vi "HFRR ADV v07 new software.vi"() -> ()   [LabVIEW 2025] (continued)
                        n2281 = local write "EVENT LOG"(w3339) -> ()
                      }
                      frame #26 {
                        n2282 = Wait (ms)(milliseconds to wait=u32 50) -> ()  [unwired: 1 out]
                      }
                      frame #27 {
                        n2283 = local read "Set Temp"() -> (w3343:dbl)
                        n2284 = Number To Fractional String(number=w3343, precision (6)=i16 2) -> (F-format string=w3344:string)  [unwired: 2 in]
                        n2285 = Concatenate Strings("Set Temperature [deg C] :" ("Content"), w3344) -> (w3346:string)
                        n2286 = local read "EVENT LOG"() -> (w3348:string)
                        n2287 = call "Event Log.vi"("Content"=w3346, "EVENT LOG"=w3348) -> ("EVENT LOG"=w3347:string)  [unwired: 8 in, 1 out]
                        n2288 = local write "EVENT LOG"(w3347) -> ()
                      }
                      frame #28 {
                        n2289 = Wait (ms)(milliseconds to wait=u32 50) -> ()  [unwired: 1 out]
                      }
                      frame #29 {
                        n2290 = local read "Set Rh"() -> (w3351:dbl)
                        n2291 = Number To Fractional String(number=w3351, precision (6)=i16 2) -> (F-format string=w3352:string)  [unwired: 2 in]
                        n2292 = Concatenate Strings("Set Humidity [%RH] :" ("Content"), w3352) -> (w3354:string)
                        n2293 = local read "EVENT LOG"() -> (w3356:string)
                        n2294 = call "Event Log.vi"("Content"=w3354, "EVENT LOG"=w3356) -> ("EVENT LOG"=w3355:string)  [unwired: 8 in, 1 out]
                        n2295 = local write "EVENT LOG"(w3355) -> ()
                      }
                      frame #30 {
                        n2296 = Wait (ms)(milliseconds to wait=u32 50) -> ()  [unwired: 1 out]
                      }
                      frame #31 {
                        n2297 = local read "test time"() -> (w3359:dbl)
                        n2298 = Number To Fractional String(number=w3359, precision (6)=i16 1) -> (F-format string=w3360:string)  [unwired: 2 in]
                        n2299 = Concatenate Strings("Test Duration [mins] :" ("Content"), w3360) -> (w3362:string)
                        n2300 = local read "EVENT LOG"() -> (w3364:string)
                        n2301 = call "Event Log.vi"("Content"=w3362, "EVENT LOG"=w3364) -> ("EVENT LOG"=w3363:string)  [unwired: 8 in, 1 out]
                        n2302 = local write "EVENT LOG"(w3363) -> ()
                      }
                      frame #32 {
                        w3365 = dbl[] [] ("History Data")
                        w3366 = cluster{"y":dbl, dbl, "y":dbl}[] [] ("History Data")
                        w3367 = FALSE ("Visible")
                        n2303 = property on="Stroke ( mm )" class="WFChart (strict)"("History Data"=w3366) -> ()  [unwired: 2 in, 2 out]
                        n2304 = property on="Humidity ( %RH )" class="WFChart (strict)"("History Data"=w3365) -> ()  [unwired: 2 in, 2 out]
                        n2305 = property on="Temperature ( Deg C )" class="WFChart (strict)"("History Data"=w3365) -> ()  [unwired: 2 in, 2 out]
                        n2306 = property on="Electrical Contact Resistance ( % )" class="WFChart (strict)"("History Data"=w3365) -> ()  [unwired: 2 in, 2 out]
                        n2307 = property on="Coefficient of Friction" class="WFChart (strict)"("History Data"=w3365) -> ()  [unwired: 2 in, 2 out]
                        n2308 = property on="Frictional Force ( N )" class="WFChart (strict)"("History Data"=w3365) -> ()  [unwired: 2 in, 2 out]
                        n2309 = property on="Coefficient of Friction" class="WFChart (strict)"("History Data"=w3365) -> ()  [unwired: 2 in, 2 out]
                        n2310 = property on="Frictional Force ( N )" class="WFChart (strict)"("History Data"=w3365) -> ()  [unwired: 2 in, 2 out]
                        n2311 = property on="Electrical Contact Resistance ( % )" class="WFChart (strict)"("History Data"=w3365) -> ()  [unwired: 2 in, 2 out]
                        n2312 = property on="Humidity ( %RH )" class="WFChart (strict)"("History Data"=w3365) -> ()  [unwired: 2 in, 2 out]
                        n2313 = property on="Stroke ( mm )" class="WFChart (strict)"("History Data"=w3366) -> ()  [unwired: 2 in, 2 out]
                        n2314 = property on="Temperature ( Deg C )" class="WFChart (strict)"("History Data"=w3365) -> ()  [unwired: 2 in, 2 out]
                        n2315 = property on="Service Password Log" class="Str"("Visible"=w3367) -> ()  [unwired: 2 in, 2 out]
                        n2316 = property on="Password 3" class="Clust (strict)"("Visible"=w3367) -> ()  [unwired: 2 in, 2 out]
                      }
                    }
                    "TEST FILE NAM,E SAVED" <- TRUE ("TEST FILE NAM,E SAVED")
                  }
                }
              }
            }
          }
        }
        n2317 = case shown="True" w2671 {
          frame False {
            n2318 = local write "tfalg"(0.0 ("tfalg")) -> ()
          }
          frame True {
            n2319 = local read "tfalg"() -> (w2816:dbl)
            n2320 = Equal?(x=w2816, y=0.0) -> (x = y?=w2817:bool)
            n2321 = case shown="True" w2817 {
              frame False {
              }
              frame True {
                n2322 = local read "Total No. of Tests"() -> (w2820:dbl)
                n2323 = local write "tfalg"(1.0 ("tfalg")) -> ()
                n2324 = local write "acq 2"(FALSE ("acq 2")) -> ()
                n2325 = Wait (ms)(milliseconds to wait=u32 200) -> ()  [unwired: 1 out]
                n2326 = Increment(x=w2820) -> (x+1=w2819:dbl)
                n2327 = local write "Total No. of Tests"(w2819) -> ()
              }
            }
          }
        }
        n2328 = local write "Test \nStatus"(w2677) -> ()
        n2329 = local write "Save"(w2677) -> ()
        n2330 = local read "Main Tab"() -> (w2634:T2)
        n2331 = case shown="True" w2658 {
          tunnel: [FALSE ("RUN") TRUE ("RUN")] -> w2657
          tunnel: [_ 1] -> w2650
          frame False {
          }
          frame True {
          }
        }
        n2332 = In Range and Coerce(upper limit=w2665, x=w2638, lower limit=w2664) -> (In Range?=w2656:bool)  [unwired: 1 out]
        n2333 = In Range and Coerce(upper limit=w2662, x=w2637, lower limit=w2663) -> (In Range?=w2654:bool)  [unwired: 1 out]
        n2334 = case shown="True" w2670 {
          frame False {
            n2335 = local read "Rt 3"() -> (w2798:bool)
            n2336 = case shown="True" w2798 {
              frame False {
              }
              frame True {
                n2337 = local write "Rt 3"(FALSE ("Rt 3")) -> ()
                n2338 = local write "Json End Flg"(TRUE ("Upld AR 2")) -> ()
              }
            }
            "Rt" <- TRUE ("Rt")
            "Rt 2" <- FALSE ("Rt")
          }
          frame True {
            n2339 = local read "Rt"() -> (w2805:bool)
            n2340 = local write "Rt 2"(TRUE ("Rt 2")) -> ()
            n2341 = case shown="True" w2805 {
              frame False {
              }
              frame True {
                w2806 = TRUE ("Upld AR 2")
                n2342 = local write "Rt"(FALSE ("Rt")) -> ()
                n2343 = local write "Upld AR"(w2806) -> ()
                n2344 = local write "Json St Flg"(w2806) -> ()
              }
            }
            "Rt 3" <- TRUE ("Rt 3")
          }
        }
        n2345 = case shown="True" w2656 {
          tunnel: [FALSE ("RUN") TRUE ("RUN")] -> w2655
          tunnel: [_ 2] -> w2649
          frame False {
          }
          frame True {
          }
        }
        n2346 = case shown="True" w2654 {
          tunnel: [FALSE ("RUN") TRUE ("RUN")] -> w2653
          tunnel: [_ 3] -> w2648
          frame False {
          }
          frame True {
          }
        }
        n2347 = case shown="\"Acquire\"" w2634 {
          tunnel: w2636 -> [_ w2867]
          frame Default {
            w2866 = 0.0 ("output")
            n2348 = local write "PID-out"(w2866) -> ()
            n2349 = local write "Frequency ( Hz )"(w2866) -> ()
          }
          frame "Acquire" {
            n2350 = stacked-sequence {
              frame #0 {
                n2351 = local read "Auto Start Test"() -> (w2869:bool)
                n2352 = case shown="True" w2869 {
                  tunnel: "RUN" -> [w2890 w2893]
                  tunnel: [w2890 w2892] -> w2870
                  frame False {
                  }
                  frame True {
                    n2353 = local read "Auto Start Temp"() -> (w2891:bool)
                    n2354 = Or(x=w2893, y=w2891) -> (x .or. y?=w2892:bool)
                  }
                }
                n2355 = local read "clk"() -> (w2889:dbl)
                n2356 = local read "Save"() -> (w2885:bool)
                n2357 = Equal?(x=w2889, y=0.0) -> (x = y?=w2886:bool)
                n2358 = And(x=w2886, y=w2885) -> (x .and. y?=w2887:bool)
                n2359 = Not(x="Engage") -> (.not. x?=w2876:bool)
                n2360 = case shown="False" w2870 {
                  tunnel: [0.0 w2911] -> w2872
                  frame False {
                    (unwired) TRUE ("Visible")
                    n2361 = local read "Auto Start Test"() -> (w2897:bool)
                    n2362 = local write "Start Time"(TRUE ("Start Time")) -> ()
                    n2363 = property on="Stroke 2" class="DigNum (strict)"("Visible"=FALSE) -> ()  [unwired: 2 in, 2 out]
                    n2364 = case shown="False" w2897 {
                      frame False {
                        n2365 = property on="Heater Button" class="Bool (strict)"("DisabledEnum"=T15."Enabled" ("Disabled")) -> ()  [unwired: 2 in, 2 out]
                        n2366 = property on="Humidity" class="Bool (strict)"("DisabledEnum"=T15."Enabled" ("Disabled")) -> ()  [unwired: 2 in, 2 out]
                      }
                      frame True {
                      }
                    }
                    n2367 = case shown="False" "TestCompFlg" {
                      frame False {
                        n2368 = local read "StartFlg"() -> (w2905:bool)
                        n2369 = case shown="True" w2905 {
                          frame False {
                          }
                          frame True {
                            n2370 = flat-sequence {
                              frame #0 {
                                n2371 = local read "EVENT LOG"() -> (w2907:string)
                                n2372 = call "Event Log.vi"("Content"="Test was interrupted", "EVENT LOG"=w2907) -> ("EVENT LOG"=w2908:string)  [unwired: 8 in, 1 out]
                                n2373 = local write "EVENT LOG"(w2908) -> ()
                              }
                              frame #1 {
                                w2910 = FALSE ("StartFlg")
                                n2374 = property on="Heater Button" class="Bool (strict)"("Val(Sgnl)"=FALSE ("Value (Signaling)")) -> ()  [unwired: 2 in, 2 out]
                                n2375 = local write "Heater Button"(w2910) -> ()
                                n2376 = local write "StartFlg"(w2910) -> ()
                                n2377 = local write "Humidity"(w2910) -> ()
                              }
                            }
                          }
                        }
                      }
                      frame True {
                      }
                    }
                    n2378 = local write "String 14"("Test will autostart once parameters reach the set value." ("String 14")) -> ()
                  }
                  frame True {
                    (unwired) FALSE ("Visible")
                    n2379 = property on="Stroke 2" class="DigNum (strict)"("Visible"=TRUE) -> ()  [unwired: 2 in, 2 out]
                    n2380 = property on="STOP 2" class="Bool (strict)"("Disabled"=u8 2) -> ()  [unwired: 2 in, 2 out]
                    n2381 = local write "String 14"(" Running....." ("String 14")) -> ()
                    n2382 = property on="Heater Button" class="Bool (strict)"("DisabledEnum"=T15."Disabled and Grayed Out" ("Disabled")) -> ()  [unwired: 2 in, 2 out]
                    n2383 = property on="Humidity" class="Bool (strict)"("DisabledEnum"=T15."Disabled and Grayed Out" ("Disabled")) -> ()  [unwired: 2 in, 2 out]
                    n2384 = case shown="True" "Start Time" {
                      selector: "Start Time" -> [_ w2930]
                      frame False {
                      }
                      frame True {
                        n2385 = Not(x=w2930) -> (.not. x?=w2929:bool)
                        n2386 = local write "Start Time"(w2929) -> ()
                        n2387 = local read "EVENT LOG"() -> (w2931:string)
                        n2388 = call "Event Log.vi"("Content"="Test in progress", "EVENT LOG"=w2931) -> ("EVENT LOG"=w2933:string)  [unwired: 8 in, 1 out]
                        n2389 = local write "EVENT LOG"(w2933) -> ()
                      }
                    }
                    n2390 = disable-structure shown="Enabled" {
                      disable-tunnel: [w2922 w2928] -> w2911
                      frame Disabled {
                        n2391 = local read "Set Hz"() -> (w2925:dbl)
                        n2392 = call <vilib>:"Uniform White Noise Waveform.vi"() -> ("signal out"=w2924:waveform(dbl))  [unwired: 10 in, 1 out]
                        n2393 = Random Number (0-1)() -> (number: 0 to 1=w2921:dbl)
                        n2394 = Add(x=w2925, y=w2924) -> (x+y=w2923:waveform(dbl))
                        n2395 = Multiply(x=ext 0.01 ("y"), y=w2921) -> (x*y=w2919:ext)
                        n2396 = Multiply(x=w2923, y=w2919) -> (x*y=w2922:waveform(ext))
                      }
                      frame Enabled {
                        n2397 = call-poly <vilib>:"Random Number (Range).vi"("lower bound (0)"=49.5, "upper bound (100)"=50.5) -> ("number"=w2928:dbl)  [unwired: 9 in]
                      }
                    }
                    "StartFlg" <- TRUE ("StartFlg")
                  }
                }
                n2398 = case shown="True" w2887 {
                  frame False {
                  }
                  frame True {
                    n2399 = local write "clk"(10.0 ("clk")) -> ()
                    n2400 = Get Date/Time In Seconds() -> (seconds since 1Jan1904=w2936:timestamp)
                    n2401 = To Double Precision Float(number=w2936) -> (double precision float=w2934:dbl)
                    n2402 = local write "acq timer"(w2934) -> ()
                    n2403 = local write "act save time"(w2934) -> ()
                  }
                }
                n2404 = call "Elapsed Time"("Time Target (s)"="Countdown", "Reset"=w2876) -> ("Elapsed Time (s)"=w2881:dbl, "Time has Elapsed"=w2879:bool)  [unwired: 10 in, 6 out]
                "Countdown 2" <- w2881
                n2405 = Subtract(x=w2881, y=2.0) -> (x-y=w2884:dbl)
                n2406 = Less?(x=w2884, y="Countdown") -> (x < y?=w2882:bool)
                n2407 = And(x=w2882, y=w2879) -> (x .and. y?=w2878:bool)
                n2408 = case shown="True" w2878 {
                  frame False {
                  }
                  frame True {
                    (unwired) dbl[] [] ("History Data")
                    n2409 = local write "Engage"(FALSE ("Engage")) -> ()
                    n2410 = local write "RUN"(TRUE ("RUN")) -> ()
                    n2411 = local read "Humidity ( %RH )"() -> (→"Rh Before":dbl)
                  }
                }
                n2412 = local read "Test \nStatus"() -> (w2874:bool)
                n2413 = Select(t=w2872, s=w2874, f=0.0) -> (s? t:f=w2873:dbl)
                n2414 = local write "Frequency ( Hz )"(w2873) -> ()
              }
              frame #1 {
                w2959 = 1000000.0 ("x")
                # "HC;1/0\nST;VALUE"
                # "Elapsed time\ncof\nstroke\nAir temp\nTemp\nHumidity"
                # "acq timer\n\nact save time"
                # "convert to microseconds"
                n2415 = local read "COUNT"() -> (w2942:i32)
                n2416 = local read "Rate"() -> (w2955:dbl)
                n2417 = Divide(x=w2959, y=w2955) -> (x/y=w2960:dbl)
                n2418 = Greater Or Equal?(x=w2942, y=250) -> (x >= y?=w2941:bool)
                n2419 = Get Date/Time In Seconds() -> (seconds since 1Jan1904=w2962:timestamp)
                n2420 = case shown="True" w2941 {
                  frame False {
                    n2421 = local read "COUNT"() -> (w2963:i32)
                    n2422 = Increment(x=w2963) -> (x+1=w2964:i32)
                    n2423 = local write "COUNT"(w2964) -> ()
                  }
                  frame True {
                    n2424 = local write "COUNT"(0 ("COUNT")) -> ()
                  }
                }
                n2425 = local read "Samplingtime 2"() -> (w2940:dbl)
                n2426 = local read "act save time"() -> (w2957:dbl)
                n2427 = Divide(x=w2960, y=w2959) -> (x/y=w2958:dbl)
                n2428 = To Double Precision Float(number=w2962) -> (double precision float=w2951:dbl)
                n2429 = Add(x=w2957, y=w2940) -> (x+y=w2956:dbl)
                n2430 = local read "acq timer"() -> (w2961:dbl)
                n2431 = local read "COUNT"() -> (w2944:i32)
                n2432 = Greater Or Equal?(x=w2951, y=w2956) -> (x >= y?=w2939:bool)
                n2433 = Multiply(x=w2958, y=w2944) -> (x*y=w2950:dbl)
                n2434 = Subtract(x=w2951, y=w2961) -> (x-y=w2953:dbl)
                n2435 = local read "Save"() -> (w2954:bool)
                n2436 = Add(x=w2953, y=w2950) -> (x+y=w2937:dbl)
                "Elapsed time 3" <- w2937
                n2437 = And(x=w2939, y=w2954) -> (x .and. y?=w2952:bool)
                n2438 = Divide(x=w2937, y=60.0) -> (x/y=w2948:dbl)
                n2439 = local read "Test \nStatus"() -> (w2938:bool)
                n2440 = local read "clk"() -> (w2945:dbl)
                n2441 = Equal?(x=w2945, y=10.0) -> (x = y?=w2947:bool)
                n2442 = case shown="True" w2952 {
                  tunnel: w2951 -> [_ w3073]
                  tunnel: [FALSE ("Boolean 2") TRUE ("Boolean 2")] -> _
                  frame False {
                  }
                  frame True {
                    w3027 = ";" ("Substring")
                    # "Pid out/\nFreq response value"
                    n2443 = local write "act save time"(w3073) -> ()
                    n2444 = local read "FILE"() -> (w3021:string)
                    n2445 = call "file check.vi"("file name in"=w3021) -> ("error out"=w3024:errorcluster, "file name out"=w3019:string)  [unwired: 9 in]
                    n2446 = call "FILE PATH CREATION.vi"("error in"=w3024, "FILE NAME :"=w3019) -> ("FILE OUT"=w3022:path)  [unwired: 8 in, 1 out]
                    n2447 = Concatenate Strings(w3019, ".dgf" ("Substring")) -> (w3023:string)
                    n2448 = local read "FF 2"() -> (→"Frictional Force ( N )" →"Frictional Force ( N )":dbl)
                    n2449 = Build Path(base path=w3022, name or relative path=w3023) -> (appended path=w3018:path)
                    n2450 = local read "COF 2"() -> (w3032:dbl)
                    "cof" <- w3032
                    "Coefficient of Friction" <- w3032
                    "COF 4" <- w3032
                    "Coefficient of Friction" <- w3032
                    n2451 = local read "LVDT STROKE"() -> (w3016:dbl)
                    n2452 = local read "Add up Stroke"() -> (w3014:dbl)
                    n2453 = local read "TEMP"() -> (w3035:dbl)
                    "Temp" <- w3035
                    "Temperature ( Deg C )" <- w3035
                    n2454 = local read "Humidity ( %RH )"() -> (w3034:dbl)
                    "Humidity ( %RH )" <- w3034
                    "Humidity ( %RH )" <- w3034
                    n2455 = local read "Frequency ( Hz )"() -> (w3041:dbl)
                    n2456 = local read "Elapsed time"() -> (w3066:dbl)
                    n2457 = local read "AIR TEMP"() -> (w3039:dbl)
                    n2458 = local read "PID-out"() -> (w3044:dbl)
                    n2459 = Subtract(x=w3016, y=w3014) -> (x-y=w3015:dbl)
                    n2460 = Absolute Value(x=w3015) -> (abs(x)=w3013:dbl)
                    n2461 = local write "Temperature ( Deg C )"(w3035) -> ()
                    n2462 = Number To Fractional String(number=w3013, width (-)=i16 9 ("precision (6)"), precision (6)=i16 6) -> (F-format string=w3059:string)  [unwired: 1 in]
                    n2463 = Number To Fractional String(number=w3039, width (-)=i16 9 ("precision (6)"), precision (6)=i16 3) -> (F-format string=w3058:string)  [unwired: 1 in]
                    n2464 = Number To Fractional String(number=w3035, width (-)=i16 9 ("precision (6)"), precision (6)=i16 3) -> (F-format string=w3055:string)  [unwired: 1 in]
                    n2465 = Number To Fractional String(number=w3034, width (-)=i16 9 ("precision (6)"), precision (6)=i16 3) -> (F-format string=w3052:string)  [unwired: 1 in]
                    n2466 = Number To Fractional String(number=0.0, width (-)=i16 9 ("precision (6)"), precision (6)=i16 3) -> (F-format string=w3049:string)  [unwired: 1 in]
                    n2467 = Number To Fractional String(number=w3044, width (-)=i16 9 ("precision (6)"), precision (6)=i16 3) -> (F-format string=w3045:string)  [unwired: 1 in]
                    n2468 = Number To Fractional String(number=w3041, width (-)=i16 9 ("precision (6)"), precision (6)=i16 3) -> (F-format string=w3040:string)  [unwired: 1 in]
                    n2469 = Number To Fractional String(number=w3032, width (-)=i16 9 ("precision (6)"), precision (6)=i16 6) -> (F-format string=w3067:string)  [unwired: 1 in]
                    n2470 = Number To Fractional String(number=w3066, width (-)=i16 14 ("precision (6)"), precision (6)=i16 3) -> (F-format string=w3068:string)  [unwired: 1 in]
                    n2471 = Bundle("y"=1.02, w3013, "y"=0.98) -> (w3033:cluster{"y":dbl, dbl, "y":dbl})  [unwired: 1 in]
                    n2472 = Number To Fractional String(number="Ambient Humidity :", width (-)=i16 9 ("precision (6)"), precision (6)=i16 6) -> (F-format string=w3025:string)  [unwired: 1 in]
                    n2473 = local read "RUN"() -> (w3031:bool)
                    n2474 = case shown="True" w3031 {
                      tunnel: w3033 -> [_ w3078]
                      tunnel: w3013 -> [_ w3077]
                      tunnel: w3013 -> [_ w3075]
                      tunnel: w3013 -> [_ w3076]
                      frame False {
                      }
                      frame True {
                        "Stroke ( mm )" <- w3078
                        "Stroke ( mm )" <- w3078
                        "Stroke 4" <- w3077
                        "Stroke 3" <- w3075
                        "Stroke 2" <- w3076
                        "measured_stroke" <- w3075
                      }
                    }
                    n2475 = Concatenate Strings(w3068, w3027, w3067, w3027, w3059, w3027, w3058, w3027, w3055, w3027, w3052, w3027, w3049, w3027, w3045, w3027, w3040, w3027, w3025, "\r") -> (w3065:string)
                    n2476 = call <vilib>:"Write Characters To File.vi"("append to file? (new file:F)"=TRUE, "character string"=w3065, "file path (dialog if empty)"=w3018) -> ()  [unwired: 2 in, 1 out]
                    "refresh flag" <- TRUE ("refresh flag")
                  }
                }
                n2477 = case shown="True" w2938 {
                  tunnel: w2948 -> [_ w2974]
                  tunnel: w2953 -> [_ w2984]
                  tunnel: [0.0 w2980] -> _
                  tunnel: w2947 -> [_ w2979]
                  tunnel: [0.0 w2978] -> _
                  tunnel: w2937 -> [_ w2978]
                  tunnel: w2951 -> [w2967 _]
                  frame False {
                    n2478 = local write "acq timer"(w2967) -> ()
                    n2479 = local write "Test Duration Status"(0.0 ("Test Duration Status")) -> ()
                  }
                  frame True {
                    n2480 = local read "Set Hz"() -> (w2981:dbl)
                    n2481 = local write "Elapsed time"(w2974) -> ()
                    n2482 = local read "test time"() -> (w2973:dbl)
                    n2483 = Multiply(x=w2984, y=w2981) -> (x*y=w2983:dbl)
                    n2484 = case shown="False" w2979 {
                      tunnel: w2983 -> [w2985 _]
                      tunnel: [w2985 1.0] -> w2980
                      frame False {
                        n2485 = local write "Cycles elapsed"(w2985) -> ()
                      }
                      frame True {
                      }
                    }
                    n2486 = Greater?(x=w2974, y=w2973) -> (0:w2982:bool)
                    n2487 = Subtract(x=w2973, y=w2974) -> (x-y=w2972:dbl)
                    "time" <- w2972
                    n2488 = Multiply(x=w2972, y=60.0) -> (x*y=w2971:dbl)
                    n2489 = local write "Time Remaining"(w2971) -> ()
                    n2490 = local write "Remaining Time"(w2971) -> ()
                    n2491 = case shown="True" w2982 {
                      frame False {
                      }
                      frame True {
                        n2492 = stacked-sequence {
                          frame #0 {
                            w2990 = T15."Enabled" ("Disabled")
                            w2989 = FALSE ("TEST FILE NAM,E SAVED")
                            w2991 = "" ("FILE")
                            w2992 = TRUE ("Visible")
                            n2493 = local write "Humidity"(FALSE ("Humidity")) -> ()
                            n2494 = local write "RUN"(FALSE ("OK Button 2")) -> ()
                            n2495 = local write "Heater Button"(FALSE ("Heater Button")) -> ()
                            n2496 = local write "Auto Start Test"(FALSE ("Auto Start Test")) -> ()
                            n2497 = local write "TestCompFlg"(TRUE ("StpFlg")) -> ()
                            n2498 = local read "Humidity ( %RH )"() -> (→"Rh After":dbl)
                            n2499 = property on="STOP 2" class="Bool (strict)"("Disabled"=u8 0) -> ()  [unwired: 2 in, 2 out]
                            n2500 = local read "EVENT LOG"() -> (w2997:string)
                            n2501 = call "Event Log.vi"("Content"="Test Completed", "EVENT LOG"=w2997) -> ("EVENT LOG"=w2996:string)  [unwired: 8 in, 1 out]
                            n2502 = property on="RUN" class="Bool (strict)"("Visible"=w2992) -> ()  [unwired: 2 in, 2 out]
                            n2503 = property on="Auto Start Test" class="Bool (strict)"("Visible"=w2992) -> ()  [unwired: 2 in, 2 out]
                            n2504 = local write "Batch Ref Num :"(w2991) -> ()
                            n2505 = local write "FILE"(w2991) -> ()
                            n2506 = local write "EVENT LOG"(w2996) -> ()
                            n2507 = local write "TEST FILE NAM,E SAVED"(w2989) -> ()
                            n2508 = local write "Fuel Discription :"(w2991) -> ()
                            n2509 = local write "START TEMP"(w2989) -> ()
                            n2510 = local write "Remarks :"(w2991) -> ()
                            n2511 = local write "Main Dashboard Buttons"(T1."Imaging" ("Main Dashboard Buttons")) -> ()
                            n2512 = local write "Main Tab"(T2."Adv Scar" ("Main Tab")) -> ()
                            n2513 = property on="FRICVALZ 2" class="Bool (strict)"("DisabledEnum"=w2990) -> ()  [unwired: 2 in, 2 out]
                            n2514 = property on="FRICVALZ 3" class="Bool (strict)"("DisabledEnum"=w2990) -> ()  [unwired: 2 in, 2 out]
                            n2515 = property on="FRICVALZ 4" class="Bool (strict)"("DisabledEnum"=w2990) -> ()  [unwired: 2 in, 2 out]
                          }
                          frame #1 {
                            n2516 = Wait (ms)(milliseconds to wait=u32 1500) -> ()  [unwired: 1 out]
                          }
                          frame #2 {
                            n2517 = local write "Command"("VC;0") -> ()
                          }
                          frame #3 {
                            n2518 = Wait (ms)(milliseconds to wait=u32 1500) -> ()  [unwired: 1 out]
                          }
                          frame #4 {
                            n2519 = local write "Command"("VC;0") -> ()
                          }
                          frame #5 {
                            n2520 = Wait (ms)(milliseconds to wait=u32 1500) -> ()  [unwired: 1 out]
                          }
                          frame #6 {
                            n2521 = local write "Command"("ST;0") -> ()
                          }
                          frame #7 {
                            n2522 = local write "measured_stroke"(0.0 ("measured_stroke")) -> ()
                            n2523 = Wait (ms)(milliseconds to wait=u32 1500) -> ()  [unwired: 1 out]
                          }
                          frame #8 {
                            n2524 = local write "Command"("HE;0") -> ()
                          }
                        }
                      }
                    }
                    n2525 = Divide(x=w2974, y=w2973) -> (x/y=w2977:dbl)
                    n2526 = Multiply(x=w2977, y=100.0) -> (x*y=w2975:dbl)
                    n2527 = local write "Test Duration Status"(w2975) -> ()
                  }
                }
              }
              frame #2 {
                n2528 = case shown="True" "Heater Button" {
                  tunnel: [0.0 ("output") w3101] -> w3079
                  frame False {
                    w3082 = TRUE ("tmpchk")
                    n2529 = local read "TEMP"() -> (w3083:dbl)
                    n2530 = local write "Temp ini"(w3083) -> ()
                    n2531 = local write "Reset 4"(w3082) -> ()
                    n2532 = local write "tmpchk"(w3082) -> ()
                    n2533 = local write "reinit"(TRUE ("reinit")) -> ()
                    n2534 = local write "manual temp log"(TRUE ("manual temp log")) -> ()
                  }
                  frame True {
                    # "Logic to turn off\nthe heater when \ntemp is not rising.\nTime - 60 sec\nDelta t- 5°c"
                    n2535 = local read "Temp ini"() -> (w3090:dbl)
                    n2536 = local read "Auto Start Test"() -> (w3086:bool)
                    n2537 = Less?(x=w3090, y=53.0) -> (x < y?=w3088:bool)
                    n2538 = case shown="False" w3086 {
                      frame False {
                        n2539 = local read "Set Temp"() -> (w3110:dbl)
                        n2540 = local read "TEMP"() -> (w3109:dbl)
                        n2541 = Subtract(x=w3110, y=w3109) -> (x-y=w3108:dbl)
                        n2542 = Absolute Value(x=w3108) -> (abs(x)=w3107:dbl)
                        n2543 = Less?(x=w3107, y=0.5) -> (x < y?=w3105:bool)
                        n2544 = case shown="True" w3105 {
                          tunnel: "manual temp log" -> [_ w3111]
                          frame False {
                          }
                          frame True {
                            n2545 = case shown="True" w3111 {
                              selector: w3111 -> [_ w3112]
                              frame False {
                              }
                              frame True {
                                # "#Event log"
                                n2546 = Not(x=w3112) -> (.not. x?=w3113:bool)
                                n2547 = local write "manual temp log"(w3113) -> ()
                                n2548 = local read "EVENT LOG"() -> (w3116:string)
                                n2549 = call "Event Log.vi"("Content"="Target Temperature reached", "EVENT LOG"=w3116) -> ("EVENT LOG"=w3115:string)  [unwired: 8 in, 1 out]
                                n2550 = local write "EVENT LOG"(w3115) -> ()
                              }
                            }
                          }
                        }
                      }
                      frame True {
                        n2551 = local write "manual temp log"(TRUE ("manual temp log")) -> ()
                      }
                    }
                    n2552 = And(x="tmpchk", y=w3088) -> (x .and. y?=w3091:bool)
                    n2553 = case shown="True" w3091 {
                      frame False {
                      }
                      frame True {
                        n2554 = call "Elapsed Time8"("Time Target (s)"=300.0, "Reset"="Reset 4") -> ("Time has Elapsed"=w3118:bool)  [unwired: 10 in, 7 out]
                        n2555 = flat-sequence {
                          tunnel: w3118 -> [_]
                          frame #0 {
                            n2556 = local write "Reset 4"(FALSE ("Reset 4")) -> ()
                          }
                        }
                        n2557 = case shown="True" w3118 {
                          frame False {
                          }
                          frame True {
                            n2558 = local read "Temp ini"() -> (w3125:dbl)
                            n2559 = Add(x=w3125, y=5.0) -> (x+y=w3123:dbl)
                            n2560 = local read "TEMP"() -> (w3126:dbl)
                            n2561 = Greater?(x=w3126, y=w3123) -> (0:w3124:bool)
                            n2562 = case shown="False" w3124 {
                              frame False {
                                n2563 = local write "Heater Button"(FALSE ("Heater Button")) -> ()
                              }
                              frame True {
                                n2564 = local write "tmpchk"(FALSE ("tmpchk")) -> ()
                              }
                            }
                          }
                        }
                      }
                    }
                    n2565 = local read "Set Temp"() -> (w3099:dbl)
                    n2566 = local read "TEMP"() -> (w3093:dbl)
                    n2567 = call-poly <vilib>:"PID.vi"("reinitialize? (F)"="reinit", "dt (s)"=-1.0, "process variable"=w3093, "setpoint"=w3099) -> ("output"=w3096:dbl)  [unwired: 6 in, 1 out]
                    n2568 = Subtract(x=w3099, y=w3093) -> (x-y=w3100:dbl)
                    n2569 = Add(x=w3099, y=0.5) -> (x+y=w3097:dbl)
                    n2570 = Greater Or Equal?(x=w3093, y=w3097) -> ()  [unwired: 1 out]
                    n2571 = Select(t=0.0, s=FALSE, f=w3096) -> (s? t:f=w3095:dbl)
                    "PID output" <- w3095
                    n2572 = flat-sequence {
                      tunnel: w3095 -> [w3129]
                      tunnel: [w3129] -> w3101
                      frame #0 {
                        n2573 = local write "reinit"(FALSE ("reinit")) -> ()
                      }
                    }
                    n2574 = Bundle(w3100, "output"=w3095, "TEMP"=w3093) -> ()  [unwired: 1 in, 1 out]
                  }
                }
                "PID-out" <- w3079
              }
              frame #3 {
                n2575 = local read "TEMP"() -> (w3131:dbl)
                n2576 = Greater Or Equal?(x=w3131, y="Set Temp 2") -> (x >= y?=w3136:bool)
                n2577 = case shown="True" w3136 {
                  tunnel: [FALSE TRUE] -> w3134
                  frame False {
                  }
                  frame True {
                  }
                }
                "Status 13" <- w3134
                n2578 = And(x=w3134, y="trip1 8") -> (x .and. y?=w3133:bool)
                n2579 = case shown="True" w3133 {
                  frame False {
                    n2580 = local write "Heater Trip Temp"(TRUE ("Heater Trip Temp")) -> ()
                  }
                  frame True {
                    w3139 = FALSE ("OK Button 2")
                    n2581 = case shown="True" "Heater Trip Temp" {
                      selector: "Heater Trip Temp" -> [_ w3141]
                      frame False {
                      }
                      frame True {
                        n2582 = Not(x=w3141) -> (.not. x?=w3140:bool)
                        n2583 = local read "EVENT LOG"() -> (w3144:string)
                        n2584 = local write "Heater Trip Temp"(w3140) -> ()
                        n2585 = call "Event Log.vi"("Content"="Heater Trip", "EVENT LOG"=w3144) -> ("EVENT LOG"=w3143:string)  [unwired: 8 in, 1 out]
                        n2586 = local write "EVENT LOG"(w3143) -> ()
                      }
                    }
                    n2587 = local write "RUN"(w3139) -> ()
                    n2588 = property on="Auto Start Test" class="Bool (strict)"("Value"=w3139) -> ()  [unwired: 2 in, 2 out]
                    n2589 = local write "Heater Button"(w3139) -> ()
                  }
                }
              }
            }
            n2590 = case shown="False" w2867 {
              frame False {
                n2591 = disable-structure shown="Disabled" {
                  frame Disabled {
                    n2592 = stacked-sequence {
                      frame #0 {
                        n2593 = local write "RUN"(FALSE ("OK Button 2")) -> ()
                      }
                      frame #1 {
                      }
                    }
                  }
                  frame Enabled {
                  }
                }
              }
              frame True {
              }
            }
          }
        }
        n2594 = local read "airtempflg"() -> (w2659:bool)
        n2595 = Or(x=w2659, y=w2657) -> (x .or. y?=w2660:bool)
        n2596 = Insert Into Array(array=string[] ["Air Temperature has reached set value,", "Humidity has reached set value,", "Sample Temperaturehas reached set value,", ""], index=0, new element="") -> (w2645:string[])
        n2597 = Build Array(w2650, w2649, w2648) -> (w2646:i32[])
        n2598 = disable-structure shown="Disabled" {
          disable-tunnel: w2660 -> [w2737 _]
          disable-tunnel: w2655 -> [w2736 _]
          disable-tunnel: w2653 -> [w2735 _]
          frame Disabled {
            n2599 = Compound Arithmetic op=AND(w2737, w2736, w2735) -> ()  [unwired: 1 out]
            n2600 = case shown="True" {
              selector: _ -> [_ _]
              frame False {
              }
              frame True {
                w2738 = FALSE ("autostrtflg")
                n2601 = local write "RUN"(TRUE ("RUN")) -> ()
                n2602 = local write "autostrtflg"(w2738) -> ()
                n2603 = local write "autostart"(w2738) -> ()
                n2604 = local write "String 14"(" Running....." ("String 14")) -> ()
              }
            }
          }
          frame Enabled {
          }
        }
        n2605 = for {
          tunnel: w2646 -> [w2788] mode=indexing
          tunnel: w2645 -> [w2787]
          shift-right: [w2784] -> w2644
          shift-left: "" -> [w2786]
          n2606 = Index Array(array=w2787, index=w2788) -> (element=w2785:string)
          n2607 = Concatenate Strings(w2785, w2786) -> (w2784:string)
        }
        n2608 = local write "autostart 2"(w2644) -> ()
        n2609 = local read "Reset Graph"() -> (w2633:bool)
        n2610 = case shown="True" w2633 {
          selector: w2633 -> [_ w2687]
          frame False {
          }
          frame True {
            w2701 = 0.0 ("X Scale.Range:Maximum")
            n2611 = Not(x=w2687) -> (.not. x?=w2686:bool)
            n2612 = local write "Reset Graph"(w2686) -> ()
            n2613 = property on="Electrical Contact Resistance ( % )" class="WFChart (strict)"("XScale.Maximum"=600.0 ("X Scale.Range:Maximum"), "XScale.Minimum"=0.0 ("X Scale.Range:Minimum"), "YScale.Maximum"=100.0 ("Y Scale.Range:Maximum"), "YScale.Minimum"=0.0 ("Y Scale.Range:Minimum")) -> ()  [unwired: 2 in, 2 out]
            n2614 = property on="Frictional Force ( N )" class="WFChart (strict)"("XScale.Maximum"=600.0 ("X Scale.Range:Maximum"), "XScale.Minimum"=0.0 ("X Scale.Range:Minimum"), "YScale.Maximum"=100.0 ("Y Scale.Range:Maximum"), "YScale.Minimum"=0.0 ("Y Scale.Range:Minimum")) -> ()  [unwired: 2 in, 2 out]
            n2615 = property on="Temperature ( Deg C )" class="WFChart (strict)"("XScale.Maximum"=600.0 ("X Scale.Range:Maximum"), "XScale.Minimum"=0.0 ("X Scale.Range:Minimum"), "YScale.Maximum"=100.0 ("Y Scale.Range:Maximum"), "YScale.Minimum"=0.0 ("Y Scale.Range:Minimum")) -> ()  [unwired: 2 in, 2 out]
            n2616 = property on="Humidity ( %RH )" class="WFChart (strict)"("XScale.Maximum"=600.0 ("X Scale.Range:Maximum"), "XScale.Minimum"=0.0 ("X Scale.Range:Minimum"), "YScale.Maximum"=100.0 ("Y Scale.Range:Maximum"), "YScale.Minimum"=0.0 ("Y Scale.Range:Minimum")) -> ()  [unwired: 2 in, 2 out]
            n2617 = property on="Stroke ( mm )" class="WFChart (strict)"("XScale.Maximum"=600.0 ("X Scale.Range:Maximum"), "XScale.Minimum"=0.0 ("X Scale.Range:Minimum"), "YScale.Maximum"=100.0 ("Y Scale.Range:Maximum"), "YScale.Minimum"=0.0 ("Y Scale.Range:Minimum")) -> ()  [unwired: 2 in, 2 out]
            n2618 = property on="Coefficient of Friction" class="WFChart (strict)"("XScale.Maximum"=600.0 ("X Scale.Range:Maximum"), "XScale.Minimum"=0.0 ("X Scale.Range:Minimum"), "YScale.Maximum"=100.0 ("Y Scale.Range:Maximum"), "YScale.Minimum"=0.0 ("Y Scale.Range:Minimum")) -> ()  [unwired: 2 in, 2 out]
            n2619 = property on="Electrical Contact Resistance ( % )" class="WFChart (strict)"("XScale.Minimum"=0.0 ("X Scale.Range:Minimum"), "XScale.Maximum"=600.0 ("X Scale.Range:Maximum"), "YScale.Minimum"=0.0 ("Y Scale.Range:Minimum"), "YScale.Maximum"=100.0 ("Y Scale.Range:Maximum")) -> ()  [unwired: 2 in, 2 out]
            n2620 = property on="Temperature ( Deg C )" class="WFChart (strict)"("XScale.Minimum"=0.0 ("X Scale.Range:Minimum"), "XScale.Maximum"=600.0 ("X Scale.Range:Maximum"), "YScale.Minimum"=0.0 ("Y Scale.Range:Minimum"), "YScale.Maximum"=100.0 ("Y Scale.Range:Maximum")) -> ()  [unwired: 2 in, 2 out]
            n2621 = property on="Coefficient of Friction" class="WFChart (strict)"("XScale.Minimum"=0.0 ("X Scale.Range:Minimum"), "XScale.Maximum"=600.0 ("X Scale.Range:Maximum"), "YScale.Maximum"=1.0 ("X Scale.Range:Minimum"), "YScale.Minimum"=0.0 ("X Scale.Range:Minimum")) -> ()  [unwired: 2 in, 2 out]
            n2622 = property on="Frictional Force ( N )" class="WFChart (strict)"("XScale.Maximum"=600.0 ("X Scale.Range:Maximum"), "XScale.Minimum"=w2701, "YScale.Maximum"=10.0 ("Y Scale.Range:Maximum"), "YScale.Minimum"=w2701) -> ()  [unwired: 2 in, 2 out]
            n2623 = property on="Stroke ( mm )" class="WFChart (strict)"("XScale.Maximum"=600.0 ("X Scale.Range:Maximum"), "XScale.Minimum"=0.0 ("X Scale.Range:Minimum"), "YScale.Maximum"=100.0 ("Y Scale.Range:Maximum"), "YScale.Minimum"=0.0 ("Y Scale.Range:Minimum")) -> ()  [unwired: 2 in, 2 out]
            n2624 = property on="Humidity ( %RH )" class="WFChart (strict)"("XScale.Maximum"=600.0 ("X Scale.Range:Maximum"), "XScale.Minimum"=0.0 ("X Scale.Range:Minimum"), "YScale.Maximum"=100.0 ("Y Scale.Range:Maximum"), "YScale.Minimum"=0.0 ("Y Scale.Range:Minimum")) -> ()  [unwired: 2 in, 2 out]
          }
        }
      }
      frame "Compare Files" {
        # "Elapsed time\ncof\nstroke\nAir temp\nTemp\nHumidity"
        n2625 = case shown="True" "RSTV1 2" {
          frame False {
          }
          frame True {
            n2626 = property on="Humidity ( %RH )" class="XYGraph (strict)"("Y Scale.Display Format:Precision"=u8 0 ("Y Scale.Format & Precision:Precision")) -> ()  [unwired: 2 in, 2 out]
            n2627 = property on="Humidity ( %RH )" class="XYGraph (strict)"("X Scale.Range:Minimum"=0.0, "X Scale.Range:Maximum"=75.0, "Y Scale.Range:Minimum"=48.0, "Y Scale.Range:Maximum"=58.0) -> ()  [unwired: 2 in, 2 out]
          }
        }
        n2628 = case shown="True" "RST CP 2" {
          frame False {
          }
          frame True {
            n2629 = property on="XY Graph 13" class="XYGraph (strict)"("Y Scale.Display Format:Precision"=u8 0 ("Y Scale.Format & Precision:Precision")) -> ()  [unwired: 2 in, 2 out]
            n2630 = property on="XY Graph 13" class="XYGraph (strict)"("X Scale.Range:Minimum"=0.0, "X Scale.Range:Maximum"=75.0, "Y Scale.Range:Minimum"=0.0, "Y Scale.Range:Maximum"=100.0) -> ()  [unwired: 2 in, 2 out]
          }
        }
        n2631 = case shown="True" "RST CP" {
          frame False {
          }
          frame True {
            n2632 = property on="Sample Temperature ( °C )" class="XYGraph (strict)"("Y Scale.Display Format:Precision"=u8 2 ("Y Scale.Format & Precision:Precision")) -> ()  [unwired: 2 in, 2 out]
            n2633 = property on="Sample Temperature ( °C )" class="XYGraph (strict)"("X Scale.Range:Minimum"=0.0, "X Scale.Range:Maximum"=75.0, "Y Scale.Range:Minimum"=58.0, "Y Scale.Range:Maximum"=62.0) -> ()  [unwired: 2 in, 2 out]
          }
        }
        n2634 = case shown="True" "RSTV1 3" {
          frame False {
          }
          frame True {
            n2635 = property on="Air Temperature  ( °C )" class="XYGraph (strict)"("Y Scale.Display Format:Precision"=u8 2 ("Y Scale.Format & Precision:Precision")) -> ()  [unwired: 2 in, 2 out]
            n2636 = property on="Air Temperature  ( °C )" class="XYGraph (strict)"("X Scale.Range:Minimum"=0.0 ("Y Scale.Range:Minimum"), "X Scale.Range:Maximum"=75.0 ("Y Scale.Range:Maximum"), "Y Scale.Range:Minimum"=20.0 ("X Scale.Range:Minimum"), "Y Scale.Range:Maximum"=26.0 ("X Scale.Range:Maximum")) -> ()  [unwired: 2 in, 2 out]
          }
        }
        n2637 = case shown="True" "RSTV1 4" {
          frame False {
          }
          frame True {
            n2638 = property on="Stroke ( mm )" class="XYGraph (strict)"("Y Scale.Display Format:Precision"=u8 2 ("Y Scale.Format & Precision:Precision")) -> ()  [unwired: 2 in, 2 out]
            n2639 = property on="Stroke ( mm )" class="XYGraph (strict)"("X Scale.Range:Minimum"=0.0 ("Y Scale.Range:Maximum"), "X Scale.Range:Maximum"=75.0 ("X Scale.Range:Minimum"), "Y Scale.Range:Minimum"=0.98, "Y Scale.Range:Maximum"=1.02) -> ()  [unwired: 2 in, 2 out]
          }
        }
        n2640 = case shown="True" "rstv2" {
          frame False {
          }
          frame True {
            n2641 = property on="Coefficient Of Friction" class="XYGraph (strict)"("Y Scale.Display Format:Precision"=u8 3 ("Y Scale.Format & Precision:Precision")) -> ()  [unwired: 2 in, 2 out]
            n2642 = property on="Coefficient Of Friction" class="XYGraph (strict)"("X Scale.Range:Minimum"=0.0 ("Y Scale.Range:Maximum"), "X Scale.Range:Maximum"=75.0, "Y Scale.Range:Minimum"=0.0, "Y Scale.Range:Maximum"=1.0 ("X Scale.Range:Minimum")) -> ()  [unwired: 2 in, 2 out]
          }
        }
        n2643 = case shown="True" "RST CP 3" {
          frame False {
          }
          frame True {
            n2644 = property on="Air Temp ( °C ) vs Humidity ( % RH )" class="XYGraph (strict)"("X Scale.Range:Minimum"=18.0, "X Scale.Range:Maximum"=28.0 ("X Scale.Range:Minimum"), "Y Scale.Range:Minimum"=30.0 ("X Scale.Range:Minimum"), "Y Scale.Range:Maximum"=70.0 ("X Scale.Range:Minimum")) -> ()  [unwired: 2 in, 2 out]
          }
        }
        n2645 = case shown="True" "OPEN 1" {
          frame False {
          }
          frame True {
            (unwired) 0  # existing file
            w3420 = "Choose a datalog file to open"  # prompt
            n2646 = local write "OPEN 1"(FALSE ("OPEN 1")) -> ()
            n2647 = String To Path(string="C:\\LAB-IQ\\Data\\") -> (path=w3405:path)
            n2648 = File Dialog(6:"*.dgf" ("pattern"), 7:w3420, 11:w3405) -> (0:w3403:errorcluster, 3:w3411:path)  [unwired: 4 in, 2 out]
            n2649 = Unbundle(w3403) -> ()  [unwired: 3 out]
            n2650 = Strip Path(path=w3411) -> (name=w3410:string)  [unwired: 1 out]
            n2651 = Path To String(path=w3411) -> (string=w3406:string)
            "string1" <- w3406
            n2652 = Match Pattern(string=w3410, regular expression=".dgf") -> (before substring=→"String Control":string)  [unwired: 1 in, 3 out]
            n2653 = Match Pattern(string=w3406, regular expression=".dgf" ("substring (\"\")")) -> (before substring=w3416:string)  [unwired: 1 in, 3 out]
            n2654 = Concatenate Strings(w3416, ".duf" ("Substring")) -> (w3412:string)
            n2655 = String To Path(string=w3412) -> (path=w3417:path)
            n2656 = call <vilib>:"Read Characters From File.vi"("file path (dialog if empty)"=w3417, "start of read offset (chars.:0)"=60 ("start of read offset (chars.: 0)")) -> ("character string"=→"String Control 2":string)  [unwired: 4 in, 3 out]
          }
        }
        n2657 = case shown="True" "OPEN 2" {
          frame False {
          }
          frame True {
            (unwired) 0  # existing file
            w3438 = "Choose a datalog file to open"  # prompt
            n2658 = local write "OPEN 2"(FALSE ("OPEN 1")) -> ()
            n2659 = String To Path(string="C:\\LAB-IQ\\Data\\") -> (path=w3423:path)
            n2660 = File Dialog(6:"*.dgf" ("pattern"), 7:w3438, 11:w3423) -> (0:w3421:errorcluster, 3:w3429:path)  [unwired: 4 in, 2 out]
            n2661 = Unbundle(w3421) -> ()  [unwired: 3 out]
            n2662 = Strip Path(path=w3429) -> (name=w3427:string)  [unwired: 1 out]
            n2663 = Path To String(path=w3429) -> (string=w3424:string)
            "string1 2" <- w3424
            n2664 = Match Pattern(string=w3427, regular expression=".dgf") -> (before substring=→"String Control 3":string)  [unwired: 1 in, 3 out]
            n2665 = Match Pattern(string=w3424, regular expression=".dgf" ("substring (\"\")")) -> (before substring=w3435:string)  [unwired: 1 in, 3 out]
            n2666 = Concatenate Strings(w3435, ".duf" ("Substring")) -> (w3432:string)
            n2667 = String To Path(string=w3432) -> (path=w3430:path)
            n2668 = call <vilib>:"Read Characters From File.vi"("file path (dialog if empty)"=w3430, "start of read offset (chars.:0)"=60 ("start of read offset (chars.: 0)")) -> ("character string"=→"String Control 4":string)  [unwired: 4 in, 3 out]
          }
        }
        n2669 = case shown="True" "OPEN 3" {
          frame False {
          }
          frame True {
            (unwired) 0  # existing file
            w3456 = "Choose a datalog file to open"  # prompt
            n2670 = local write "OPEN 3"(FALSE ("OPEN 1")) -> ()
            n2671 = String To Path(string="C:\\LAB-IQ\\Data\\") -> (path=w3441:path)
            n2672 = File Dialog(6:"*.dgf" ("pattern"), 7:w3456, 11:w3441) -> (0:w3439:errorcluster, 3:w3447:path)  [unwired: 4 in, 2 out]
            n2673 = Unbundle(w3439) -> ()  [unwired: 3 out]
            n2674 = Strip Path(path=w3447) -> (name=w3445:string)  [unwired: 1 out]
            n2675 = Path To String(path=w3447) -> (string=w3442:string)
            "string1 3" <- w3442
            n2676 = Match Pattern(string=w3445, regular expression=".dgf") -> (before substring=→"String Control 5":string)  [unwired: 1 in, 3 out]
            n2677 = Match Pattern(string=w3442, regular expression=".dgf" ("substring (\"\")")) -> (before substring=w3452:string)  [unwired: 1 in, 3 out]
            n2678 = Concatenate Strings(w3452, ".duf" ("Substring")) -> (w3449:string)
            n2679 = String To Path(string=w3449) -> (path=w3453:path)
            n2680 = call <vilib>:"Read Characters From File.vi"("file path (dialog if empty)"=w3453, "start of read offset (chars.:0)"=60 ("start of read offset (chars.: 0)")) -> ("character string"=→"String Control 6":string)  [unwired: 4 in, 3 out]
          }
        }
        n2681 = case shown="True" "OPEN 4" {
          frame False {
          }
          frame True {
            (unwired) 0  # existing file
            w3474 = "Choose a datalog file to open"  # prompt
            n2682 = local write "OPEN 4"(FALSE ("OPEN 1")) -> ()
            n2683 = String To Path(string="C:\\LAB-IQ\\Data\\") -> (path=w3459:path)
            n2684 = File Dialog(6:"*.dgf" ("pattern"), 7:w3474, 11:w3459) -> (0:w3457:errorcluster, 3:w3465:path)  [unwired: 4 in, 2 out]
            n2685 = Unbundle(w3457) -> ()  [unwired: 3 out]
            n2686 = Strip Path(path=w3465) -> (name=w3463:string)  [unwired: 1 out]
            n2687 = Path To String(path=w3465) -> (string=w3460:string)
            "string1 4" <- w3460
            n2688 = Match Pattern(string=w3463, regular expression=".dgf") -> (before substring=→"String Control 7":string)  [unwired: 1 in, 3 out]
            n2689 = Match Pattern(string=w3460, regular expression=".dgf" ("substring (\"\")")) -> (before substring=w3470:string)  [unwired: 1 in, 3 out]
            n2690 = Concatenate Strings(w3470, ".duf" ("Substring")) -> (w3467:string)
            n2691 = String To Path(string=w3467) -> (path=w3471:path)
            n2692 = call <vilib>:"Read Characters From File.vi"("file path (dialog if empty)"=w3471, "start of read offset (chars.:0)"=60 ("start of read offset (chars.: 0)")) -> ("character string"=→"String Control 8":string)  [unwired: 4 in, 3 out]
          }
        }
      }
      frame "About" {
        # "Elapsed time\ncof\nstroke\nmean pos\nTemp\nHumidity"
        n2693 = disable-structure shown="Disabled" {
          frame Disabled {
            n2694 = case shown="True" "Export" {
              frame False {
              }
              frame True {
                w3496 = "                                      " ("string")
                w3498 = "\r"
                (unwired) i16 6 ("width (-)")
                w3575 = "\r"
                w3507 = "\r"
                n2695 = local write "Export"(FALSE ("Export")) -> ()
                n2696 = local read "String 29"() -> (w3544:string)
                n2697 = local read "String 34"() -> (w3532:string)
                n2698 = local read "String 35"() -> (w3527:string)
                n2699 = local read "String 37"() -> (w3523:string)
                n2700 = local read "String 36"() -> (w3520:string)
                n2701 = local read "String 38"() -> (w3517:string)
                n2702 = local read "String 39"() -> (w3514:string)
                n2703 = Match Pattern(string=w3544, regular expression=".dwm") -> (before substring=w3540:string)  [unwired: 1 in, 3 out]
                "before substring" <- w3540
                n2704 = local read "S 38"() -> (w3535:string)
                n2705 = local read "S 39"() -> (w3528:string)
                n2706 = local read "Temperature before test 2"() -> (w3564:dbl)
                n2707 = local read "Temperature after test 2"() -> (w3569:dbl)
                n2708 = local read "Humidity before test 2"() -> (w3550:dbl)
                n2709 = local read "Humidity after test 2"() -> (w3565:dbl)
                n2710 = local read "MWSD 2"() -> (w3561:dbl)
                n2711 = local read "WS1.4 2"() -> (w3577:dbl)
                n2712 = local read "HCF 2"() -> (w3573:dbl)
                n2713 = local read "AVP 2"() -> (w3562:dbl)
                n2714 = Concatenate Strings("1," ("string"), w3535) -> (w3534:string)
                n2715 = Concatenate Strings("2," ("string"), w3532) -> (w3531:string)
                n2716 = Concatenate Strings("3," ("string"), w3528) -> (w3530:string)
                n2717 = Concatenate Strings("4," ("string"), w3527) -> (w3526:string)
                n2718 = Concatenate Strings("5," ("string"), w3523) -> (w3524:string)
                n2719 = Concatenate Strings("6," ("string"), w3520) -> (w3521:string)
                n2720 = Concatenate Strings("7," ("string"), w3517) -> (w3518:string)
                n2721 = Concatenate Strings("8," ("string"), w3514) -> (w3515:string)
                n2722 = local read "Sample ID"() -> (w3582:string)
                n2723 = case shown="\"xlx\"" "Select File Type" {
                  tunnel: w3540 -> [w3585 w3587 w3589]
                  tunnel: [w3583 w3588 w3590] -> w3539
                  frame "xlx" {
